vi "VIGmentize Tool.vi"() -> ()   [LabVIEW 2026]
panel:
  in  "Type ( \"\" = guess)":string
  in  "Style":T1(ring)=enum."material"
  in  "ACTION":bool
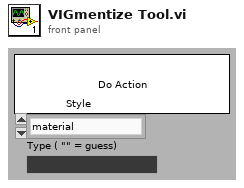
[diagram p1: front panel]
types:
  T1 = enum16{"abap", "algol", "algol_nu", "arduino", "autumn", "bw", "borland", "coffee", "colorful", "default", "dracula", "emacs", "friendly_grayscale", "friendly", "fruity", "github-dark", "gruvbox-dark", "gruvbox-light", "igor", "inkpot", "lightbulb", "lilypond", "lovelace", "manni", "material", "monokai", "murphy", "native", "nord-darker", "nord", "one-dark", "paraiso-dark", "paraiso-light", "pastie", "perldoc", "rainbow_dash", "rrt", "sas", "solarized-dark", "solarized-light", "staroffice", "stata-dark", "stata-light", "tango", "trac", "vim", "vs", "xcode", "zenburn"}
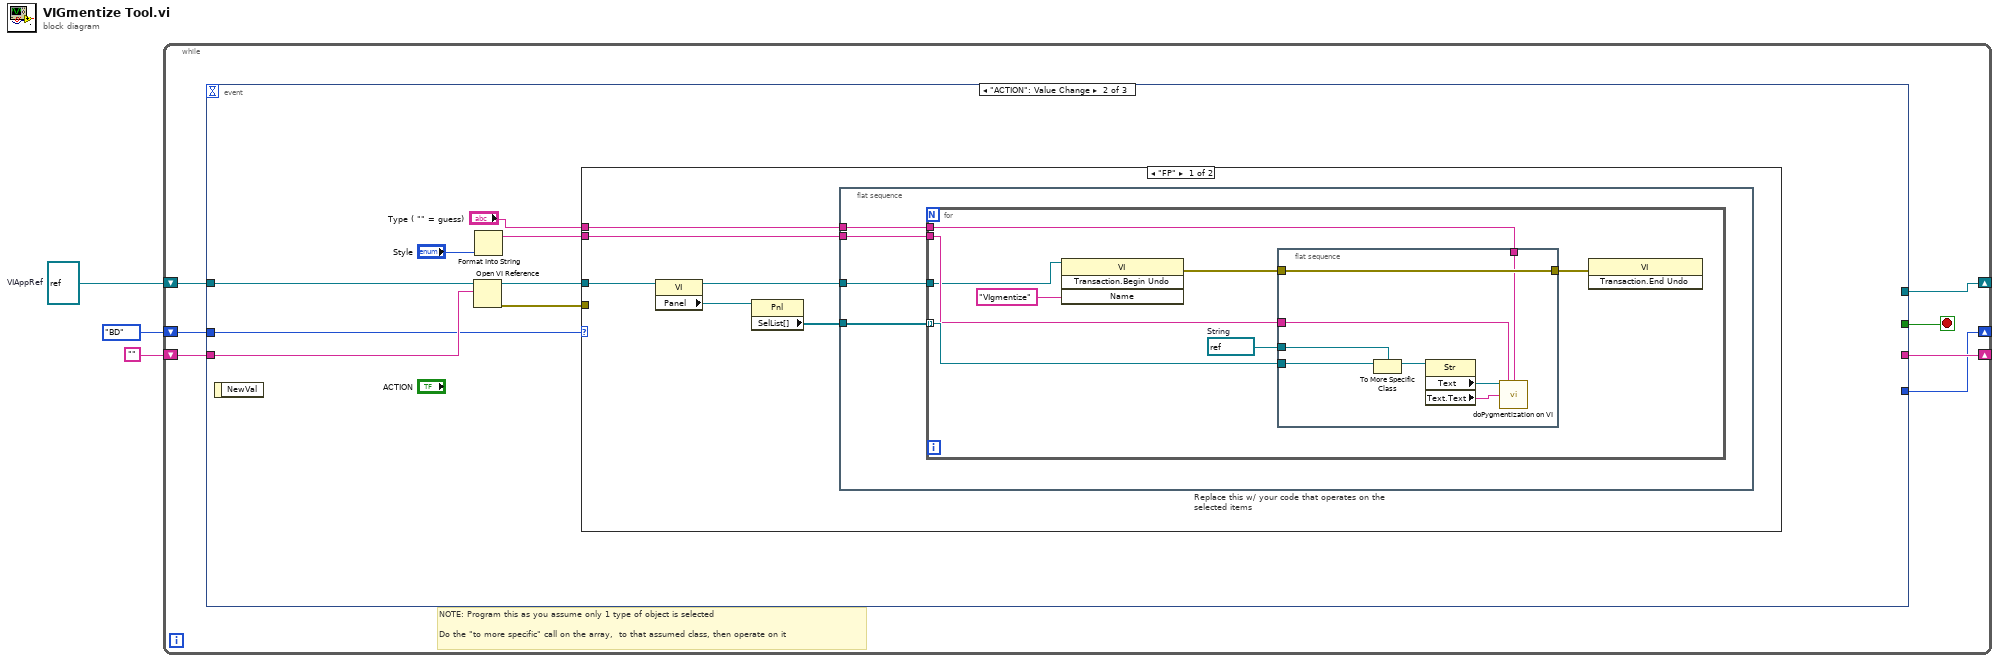
[diagram p0: block diagram]
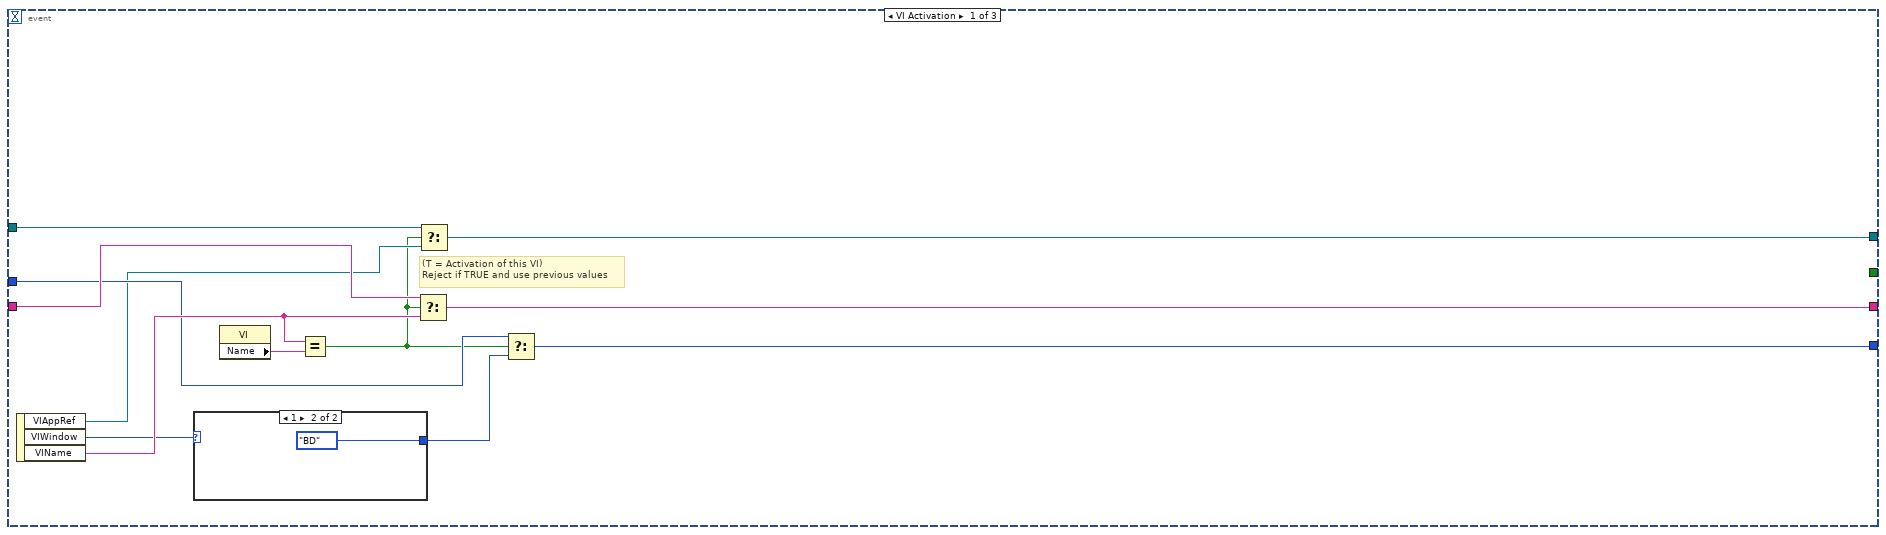
[diagram p2: hidden frame]
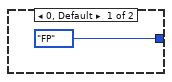
[diagram p3: hidden frame]
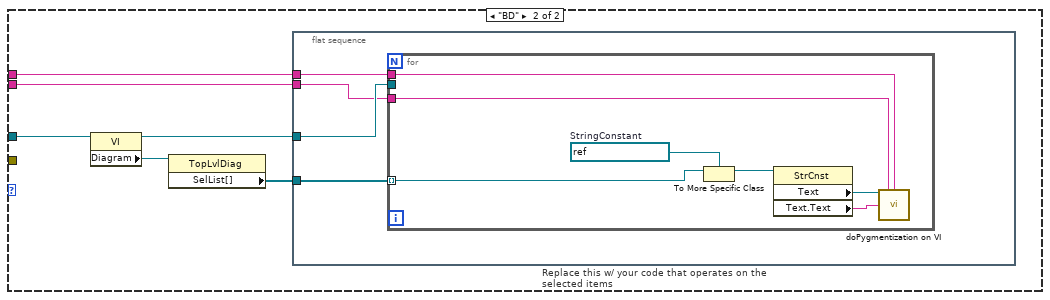
[diagram p4: hidden frame]
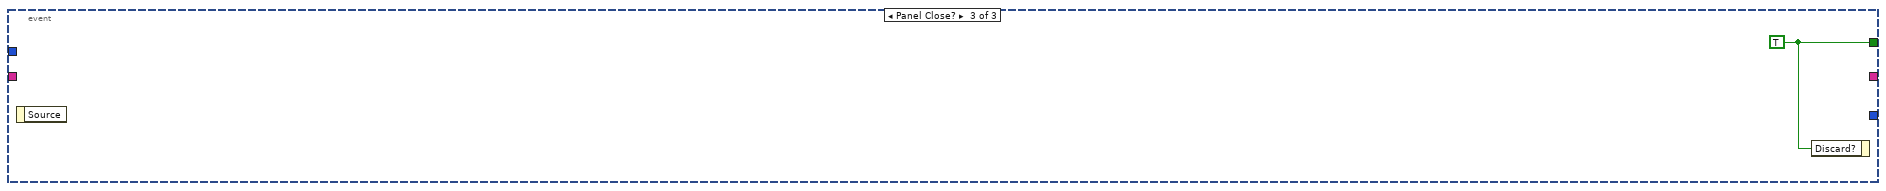
[diagram p5: hidden frame]
diagram:
  w1 = refnum<vi> refnum  # VIAppRef
  n1 = while {
    shift-right: [w10] -> _
    shift-left: "" -> [w9]
    shift-right: [w7] -> _
    shift-left: enum16{"FP", "BD"}."BD" -> [w6]
    shift-right: [w5] -> _
    shift-left: w1 -> [w4]
    stop <- w8 stop-if-true
    # "NOTE: Program this as you assume only 1 type of object is selected\n\nDo the \"to more specific\" call on the array,  to that assumed class, then operate on it"
    n2 = event shown="[1] \"ACTION\": Value Change" {
      selector: _ -> [_ _ _]
      dyn-events: _ -> [_ _ _]
      timeout: _ -> [_ _ _]
      tunnel: [w19 _ _] -> w10
      tunnel: w9 -> [w22 w32 _]
      tunnel: [_ _ w76] -> w8
      tunnel: [w17 _ _] -> w7
      tunnel: w6 -> [w18 w30 _]
      tunnel: [w13 _ _] -> w5
      tunnel: w4 -> [w12 w29 _]
      event VI Activation {
        # "(T = Activation of this VI)\nReject if TRUE and use previous values"
        n3 = event-data() -> ("VIAppRef"=w14:refnum<vi>, "VIWindow"=w16:i32, "VIName"=w20:string)  [unwired: 1 out]
        n4 = case shown="1" w16 {
          tunnel: [enum16{"FP", "BD"}."FP" enum16{"FP", "BD"}."BD"] -> w15
          frame 0, Default {
          }
          frame 1 {
          }
        }
        n5 = property class="VI"() -> ("Name"=w21:string)  [unwired: 2 in, 2 out]
        n6 = Equal?(x=w20, y=w21) -> (x = y?=w11:bool)
        n7 = Select(t=w22, s=w11, f=w20) -> (s? t:f=w19:string)
        n8 = Select(t=w12, s=w11, f=w14) -> (s? t:f=w13:refnum<vi>)
        n9 = Select(t=w18, s=w11, f=w15) -> (s? t:f=w17:enum16{"FP", "BD"})
      }
      event "ACTION": Value Change {
        n10 = event-data() -> ()  [unwired: 2 out]
        n11 = Open VI Reference(application reference (local)=w29, vi path=w32) -> (vi reference=w31:refnum<vi>, error out=w26:errorcluster)  [unwired: 2 in, 2 out]
        n12 = Format Into String("Style") -> (resulting string=w27:string)  [unwired: 3 in, 1 out]
        n13 = case shown="\"FP\"" w30 {
          tunnel: w31 -> [w38 w64]
          tunnel: w27 -> [w34 w60]
          tunnel: w26 -> [_ _]
          tunnel: "Type ( \"\" = guess)" -> [w33 w59]
          frame "FP" {
            n14 = property class="VI"(reference=w38) -> (reference out=w35:refnum<vi>, "Panel"=w37:refnum<vi>)  [unwired: 1 in, 1 out]
            n15 = property class="Pnl"(reference=w37) -> ("SelList[]"=w36:refnum<vi>[])  [unwired: 1 in, 2 out]
            n16 = flat-sequence "Replace this w/ your code that operates on the selected items" {
              tunnel: w36 -> [w42]
              tunnel: w35 -> [w41]
              tunnel: w34 -> [w40]
              tunnel: w33 -> [w39]
              frame #0 {
                n17 = for {
                  tunnel: w42 -> [w50] mode=indexing
                  tunnel: w41 -> [w47]
                  tunnel: w40 -> [w48]
                  tunnel: w39 -> [w43]
                  w49 = refnum<vi> refnum  # String
                  n18 = invoke class="VI" method="Transaction.Begin Undo"(reference=w47, "Name"="VIgmentize") -> (error out=w45:errorcluster)  [unwired: 2 in, 3 out]
                  n19 = flat-sequence {
                    tunnel: w50 -> [w58]
                    tunnel: w49 -> [w57]
                    tunnel: w48 -> [w53]
                    tunnel: w45 -> [w52]
                    tunnel: [w52] -> w44
                    tunnel: w43 -> [w51]
                    frame #0 {
                      n20 = To More Specific Class(target class=w57, reference=w58) -> (specific class reference=w56:refnum<vi>)  [unwired: 1 in, 1 out]
                      n21 = property class="Str"(reference=w56) -> ("Text"=w55:refnum<vi>, "Text.Text"=w54:string)  [unwired: 1 in, 2 out]
                      n22 = call "doPygmentization on VI.vi"("Text Field Destination"=w55, "style name (material)"=w53, "Type"=w51, "String"=w54) -> ()  [unwired: 12 in]
                    }
                  }
                  n23 = invoke class="VI" method="Transaction.End Undo"(error in=w44) -> ()  [unwired: 2 in, 3 out]
                }
              }
            }
          }
          frame "BD" {
            n24 = property class="VI"(reference=w64) -> (reference out=w61:refnum<vi>, "Diagram"=w63:refnum<vi>)  [unwired: 1 in, 1 out]
            n25 = property class="TopLvlDiag"(reference=w63) -> ("SelList[]"=w62:refnum<vi>[])  [unwired: 1 in, 2 out]
            n26 = flat-sequence "Replace this w/ your code that operates on the selected items" {
              tunnel: w62 -> [w68]
              tunnel: w61 -> [w67]
              tunnel: w60 -> [w66]
              tunnel: w59 -> [w65]
              frame #0 {
                n27 = for {
                  tunnel: w68 -> [w75] mode=indexing
                  tunnel: w67 -> [_]
                  tunnel: w66 -> [w70]
                  tunnel: w65 -> [w69]
                  w74 = refnum<vi> refnum  # StringConstant
                  n28 = To More Specific Class(target class=w74, reference=w75) -> (specific class reference=w73:refnum<vi>)  [unwired: 1 in, 1 out]
                  n29 = property class="StrCnst"(reference=w73) -> ("Text"=w72:refnum<vi>, "Text.Text"=w71:string)  [unwired: 1 in, 2 out]
                  n30 = call "doPygmentization on VI.vi"("Text Field Destination"=w72, "style name (material)"=w70, "Type"=w69, "String"=w71) -> ()  [unwired: 12 in]
                }
              }
            }
          }
        }
      }
      event Panel Close? {
        w76 = TRUE ("Discard?")
        n31 = event-data() -> ()  [unwired: 2 out]
        n32 = event-data("Discard?"=w76) -> ()  [unwired: 1 in, 1 out]
      }
    }
  }
